vi "read voltage map.vi"(8 "error in (no error)":errorcluster, 11 "BMC in":refnum<class "BMC.lvclass">) -> (0 "error out":errorcluster, 2 "1x160 Voltage Map":dbl[](array[numeric]), 3 "BMC out":refnum<class "BMC.lvclass">)   [LabVIEW 2012, in "BMC.lvclass"]
uses:
  BMC.lvclass
  BMC.lvclass/BMC.ctl
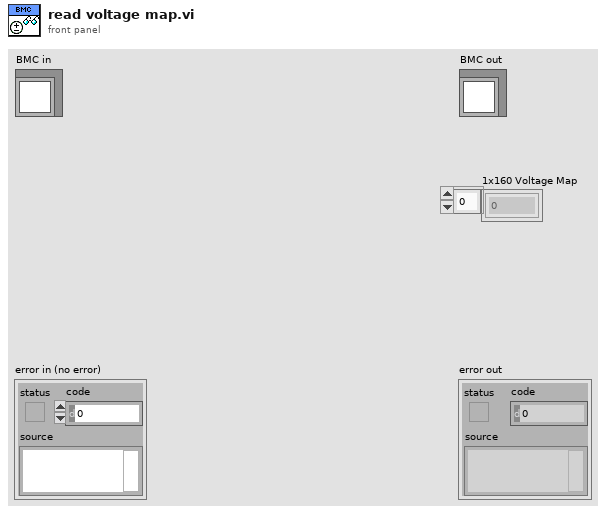
[diagram p1: front panel]
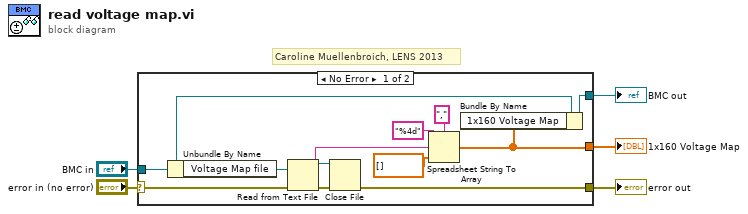
[diagram p0: block diagram]
diagram:
  # "Caroline Muellenbroich, LENS 2013"
  n1 = case shown="No Error" "error in (no error)" {
    selector: "error in (no error)" -> [w11 w19]
    tunnel: [w9 w19] -> w4
    tunnel: [w12 w18] -> w2
    tunnel: "BMC in" -> [w13 w18]
    tunnel: [w7 _] -> w1
    frame No Error {
      n2 = Unbundle By Name(w13) -> ("Voltage Map file"=w6:path)
      n3 = Read from Text File(file (use dialog)=w6, error in=w11) -> (refnum out=w14:refnum<file>, text=w17:string, error out=w10:errorcluster)  [unwired: 3 out]
      n4 = Close File(refnum=w14, error in=w10) -> (error out=w9:errorcluster)  [unwired: 1 out]
      n5 = Spreadsheet String To Array(delimiter (Tab)=",", format string="%4d", spreadsheet string=w17, array type (2D Dbl)=dbl[] [] ("run time Cluster.1x160  Voltage Map")) -> (array=w7:dbl[])
      n6 = Bundle By Name(cluster=w13, "1x160 Voltage Map"=w7) -> (w12:refnum<class "BMC.lvclass">)
    }
    frame Error {
    }
  }
  "error out" <- w4
  "BMC out" <- w2
  "1x160 Voltage Map" <- w1
